vi "HAB Climber.vi"   [LabVIEW 2018]
uses:
  <vilib>/Rock Robotics/SystemInterfaces/DIO/FPGA_DIOChannel.ctl
  <vilib>/Rock Robotics/WPI/ThirdParty/Phoenix-LabVIEW/Motor Controller/Controls/CTRE_Phoenix_MotorControl_ControlMode.ctl
  HAB Climber Global.vi
  <vilib>/Rock Robotics/WPI/Switch/WPI_SwitchOpenLimit.vi
  <vilib>/Rock Robotics/WPI/Counter/WPI_CounterDigitalInputToDigitalSource.vi
  Times/Times Global.vi
  Cargo Intake/Cargo Intake Global.vi
  Controllers/Driver Controller/Driver Controller Global.vi
types:
  T1 = typedef "FPGA_DIOChannel.ctl" = enum8{"DIO 0", "DIO 1", "DIO 2", "DIO 3", "DIO 4", "DIO 5", "DIO 6", "DIO 7", "DIO 8", "DIO 9", "DIO MXP 0", "DIO MXP 1", "DIO MXP 2", "DIO MXP 3", "DIO MXP 4", "DIO MXP 5", "DIO MXP 6", "DIO MXP 7", "DIO MXP 8", "DIO MXP 9", "DIO MXP 10", "DIO MXP 11", "DIO MXP 12", "DIO MXP 13", "DIO MXP 14", "DIO MXP 15", "SPI Port CS1", "SPI Port CS2", "SPI Port CS3", "SPI Port MISO", "SPI Port MOSI", "Invalid"}
  T2 = enum16{"HAB Climber Full Manual Mode", "HAB Climber Manual Mode", "HAB Climber Automated Mode", "HAB Climber Fully Automated Mode"}
  T3 = typedef "WPI_DigitalInputDevRef.ctl" = cluster{"DevStatus":errorcluster, "DIO Channel":T1}
  T4 = typedef "FPGA_CounterEncoderSourceConvertionLVSourceType.ctl" = cluster{"DevStatus":errorcluster, "AnalogTriggerMode?":bool, "DigitalMode":cluster{"DIO Channel":T5}, "AnalogTriggerMode":cluster{"AnalogTriggerIndex":T6, "OutputType":T7}}
  T5 = typedef "FPGA_DIODigitalSourceChannel.ctl" = enum8{"DIO 0", "DIO 1", "DIO 2", "DIO 3", "DIO 4", "DIO 5", "DIO 6", "DIO 7", "DIO 8", "DIO 9", "DIO MXP 0", "DIO MXP 1", "DIO MXP 2", "DIO MXP 3", "DIO MXP 4", "DIO MXP 5", "DIO MXP 6", "DIO MXP 7", "DIO MXP 8", "DIO MXP 9", "DIO MXP 10", "DIO MXP 11", "DIO MXP 12", "DIO MXP 13", "DIO MXP 14", "DIO MXP 15", "SPI Port CS1", "SPI Port CS2", "SPI Port CS3", "SPI Port MISO", "SPI Port MOSI", "Disabled"}
  T6 = typedef "FPGA_AnalogTriggerIndex.ctl" = enum8{"Trig 0", "Trig 1", "Trig 2", "Trig 3", "Trig 4", "Trig 5", "Trig 6", "Trig 7", "Invalid"}
  T7 = typedef "FPGA_AnalogTriggerOutType.ctl" = enum16{"InWindow", "TriggerState", "Rising", "Falling"}
  T8 = typedef "WPI_EncoderDevRef.ctl" = cluster{"DevStatus":errorcluster, "EncoderIndex":T9, "CounterIndex":T10, "DistancePerCount":dbl, "Decoding Type":T11}
  T9 = typedef "FPGA_EncoderIdx.ctl" = enum8{"Enc 0", "Enc 1", "Enc 2", "Enc 3", "Enc 4", "Enc 5", "Enc 6", "Enc 7", "Invalid"}
  T10 = typedef "FPGA_CounterCtrSystemIndex.ctl" = enum8{"Ctr 0", "Ctr 1", "Ctr 2", "Ctr 3", "Ctr 4", "Ctr 5", "Ctr 6", "Ctr 7", "Invalid"}
  T11 = typedef "WPI_EncoderType.ctl" = enum16{"1x", "2x", "4x"}
  T12 = typedef "WPI_SwitchDevRef.ctl" = cluster{"DevStatus":errorcluster, "DIO Channel":T1, "CntIndex":T10, "Normally Closed":bool}
  T13 = typedef "WPI_MotorControlDeviceRef.ctl" = cluster{"DeviceStatus":errorcluster, "Type":T14, "PWM":cluster{"PWM Channel":T15, "DeadBand":T16}, "CAN":cluster{"Device Number":u8, "SetOutput VI Ref":variant, "GetOutput VI Ref":variant, "Enable VI Ref":variant, "Disable VI Ref":variant, "Data":variant}, "Invert":bool, "DIO PWM":cluster{"PWM \"Enable\" Channel":T15, "DIOChannel":T1, "PWM Rate":dbl}}
  T14 = typedef "WPI_MotorControlType.ctl" = enum16{"PWM", "CAN", "DIO PWM"}
  T15 = typedef "FPGA_DIOPWMChannel.ctl" = enum8{"PWM 0", "PWM 1", "PWM 2", "PWM 3", "PWM 4", "PWM 5", "PWM 6", "PWM 7", "PWM 8", "PWM 9", "PWM MXP 0", "PWM MXP 1", "PWM MXP 2", "PWM MXP 3", "PWM MXP 4", "PWM MXP 5", "PWM MXP 6", "PWM MXP 7", "PWM MXP 8", "PWM MXP 9", "Invalid"}
  T16 = typedef "WPI_PWMDeadband.ctl" = cluster{"Name":string, "maxPositivePwm":i32, "minPositivePwm":i32, "centerPwm":i32, "maxNegativePwm":i32, "minNegativePwm":i32, "angularRange":u16}
  T17 = typedef "Control 3.ctl" = dbl
  T18 = typedef "CTRE_Phoenix_MotorControl_ControlMode.ctl" = u16
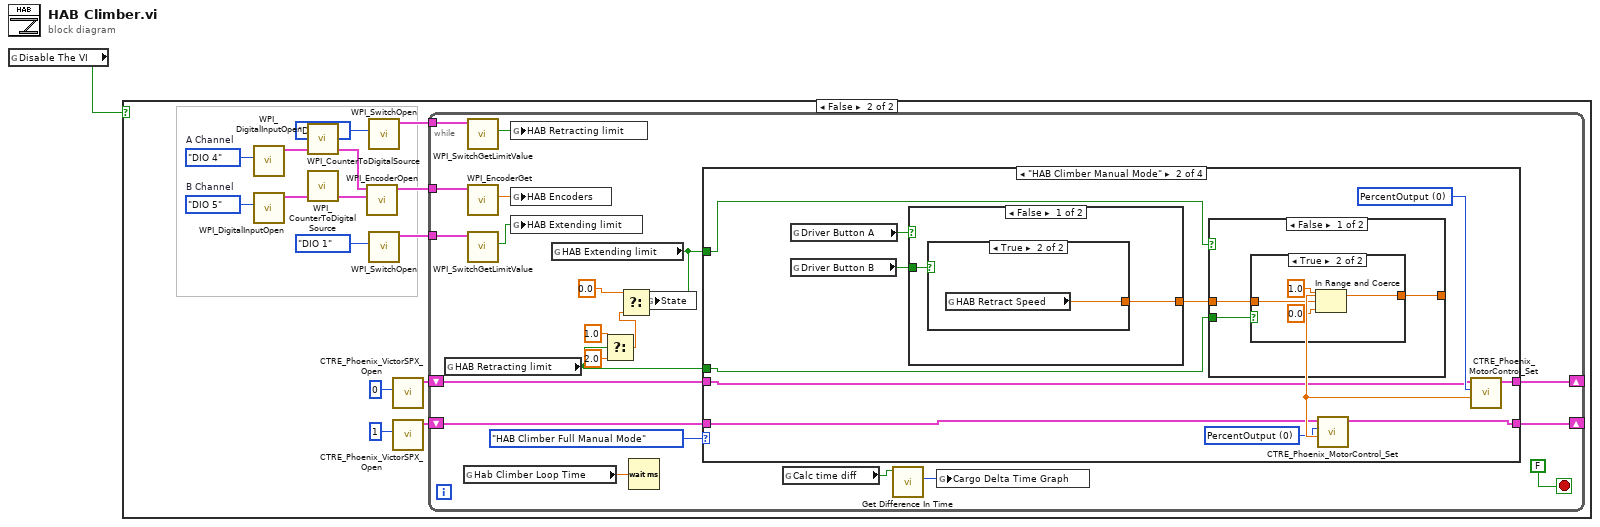
[diagram p0: block diagram]
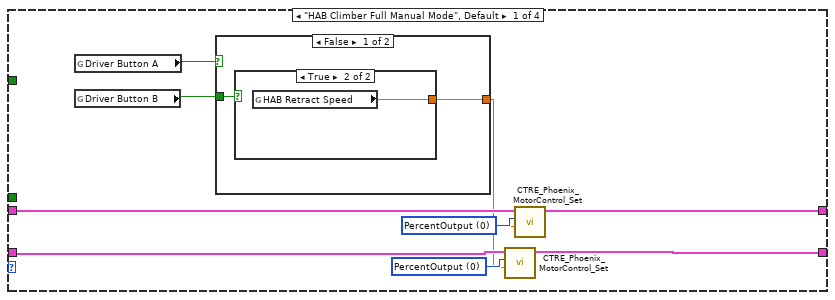
[diagram p3: hidden frame]
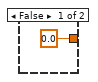
[diagram p4: hidden frame]
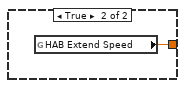
[diagram p5: hidden frame]
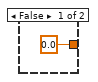
[diagram p6: hidden frame]
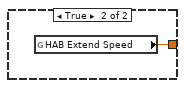
[diagram p7: hidden frame]
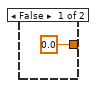
[diagram p8: hidden frame]
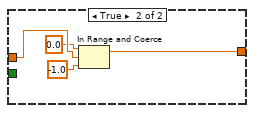
[diagram p9: hidden frame]
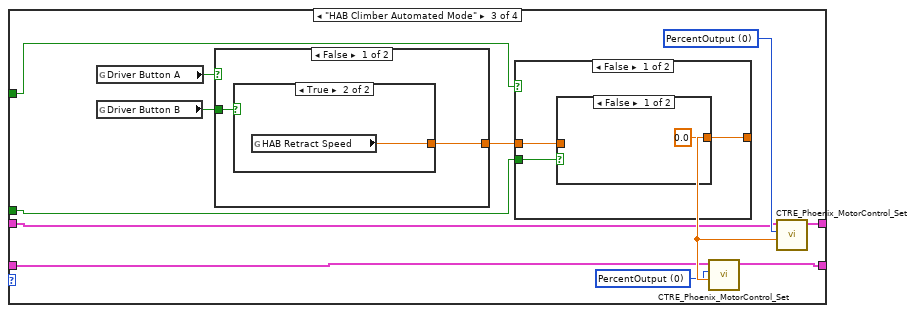
[diagram p10: hidden frame]
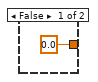
[diagram p11: hidden frame]
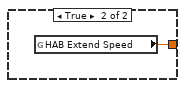
[diagram p12: hidden frame]
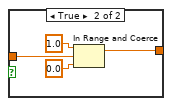
[diagram p13: hidden frame]
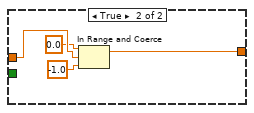
[diagram p14: hidden frame]
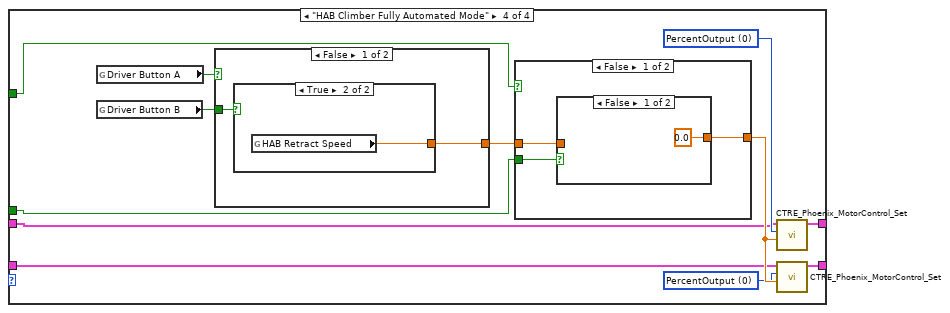
[diagram p15: hidden frame]
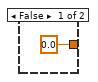
[diagram p16: hidden frame]
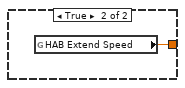
[diagram p17: hidden frame]
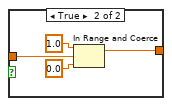
[diagram p18: hidden frame]
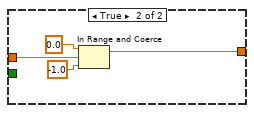
[diagram p19: hidden frame]
diagram:
  n1 = global read "HAB Climber Global.vi" "Disable The VI"() -> (w1:bool)
  n2 = case shown="False" w1 {
    frame True {
    }
    frame False {
      w8 = FPGA_DIOChannel."DIO 5"  # B Channel
      w7 = FPGA_DIOChannel."DIO 4"  # A Channel
      n3 = call <vilib>:"WPI_DigitalInputOpen.vi"("DIO Channel"=w7) -> ("DigitalInputDevRef"=w4:T3)  [unwired: 1 in, 9 out]
      n4 = call <vilib>:"WPI_DigitalInputOpen.vi"("DIO Channel"=w8) -> ("DigitalInputDevRef"=w5:T3)  [unwired: 1 in, 9 out]
      n5 = call-poly <vilib>:"WPI_CounterToDigitalSource.vi"("DigitalInputDevRef"=w4) -> ("Digital Source"=w3:T4)  [unwired: 6 out]
      n6 = call-poly <vilib>:"WPI_CounterToDigitalSource.vi"("DigitalInputDevRef"=w5) -> ("Digital Source"=w6:T4)  [unwired: 6 out]
      n7 = call <vilib>:"WPI_EncoderOpen.vi"("BSource"=w6, "ASource"=w3) -> ("EncoderDevRef"=w2:T8)  [unwired: 6 in, 3 out]
      n8 = call-poly <vilib>:"WPI_SwitchOpen.vi"("DIO Channel"=FPGA_DIOChannel."DIO 2") -> ("SwitchDevRef"=w10:T12)  [unwired: 9 in, 1 out]
      n9 = call-poly <vilib>:"WPI_SwitchOpen.vi"("DIO Channel"=FPGA_DIOChannel."DIO 1") -> ("SwitchDevRef"=w9:T12)  [unwired: 9 in, 1 out]
      n10 = call <vilib>:"CTRE_Phoenix_VictorSPX_Open.vi"("Device Number"=u8 0) -> ("CAN Talon SRX Ref"=w16:T13)  [unwired: 9 in, 1 out]
      n11 = call <vilib>:"CTRE_Phoenix_VictorSPX_Open.vi"("Device Number"=u8 1) -> ("CAN Talon SRX Ref"=w14:T13)  [unwired: 9 in, 1 out]
      n12 = while {
        shift-right: [w33] -> _
        shift-left: w16 -> [w35]
        shift-right: [w32] -> _
        shift-left: w14 -> [w34]
        tunnel: w10 -> [w25]
        tunnel: w9 -> [w24]
        tunnel: w2 -> [w23]
        stop <- FALSE stop-if-true
        n13 = global read "HAB Climber Global.vi" "HAB Retracting limit"() -> (w21:bool)
        n14 = global read "Times Global.vi" "Hab Climber Loop Time"() -> (w38:T17)
        n15 = call <vilib>:"WPI_SwitchGetLimitValue.vi"("SwitchDevRef"=w25) -> ("Switch Pressed"=w19:bool)  [unwired: 8 in, 2 out]
        n16 = call <vilib>:"WPI_EncoderGet.vi"("EncoderDevRef"=w23) -> ("Distance"=w18:dbl)  [unwired: 5 in, 5 out]
        n17 = call <vilib>:"WPI_SwitchGetLimitValue.vi"("SwitchDevRef"=w24) -> ("Switch Pressed"=w20:bool)  [unwired: 8 in, 2 out]
        n18 = global write "HAB Climber Global.vi" "HAB Retracting limit"(w19) -> ()
        n19 = global write "HAB Climber Global.vi" "HAB Encoders"(w18) -> ()
        n20 = global write "HAB Climber Global.vi" "HAB Extending limit"(w20) -> ()
        n21 = global read "HAB Climber Global.vi" "HAB Extending limit"() -> (w22:bool)
        n22 = Select(t=1.0, s=w21, f=2.0 ("t")) -> (s? t:f=w17:dbl)
        n23 = Select(t=0.0, s=w22, f=w17) -> (s? t:f=w29:dbl)
        n24 = Wait (ms)(milliseconds to wait=w38) -> ()  [unwired: 1 out]
        n25 = global write "HAB Climber Global.vi" "State"(w29) -> ()
        n26 = case shown="\"HAB Climber Manual Mode\"" T2."HAB Climber Full Manual Mode" ("Mode") {
          tunnel: w35 -> [w42 w58 w87 w116]
          tunnel: w34 -> [w43 w57 w86 w115]
          tunnel: [w40 w56 w85 w114] -> w33
          tunnel: [w39 w55 w84 w113] -> w32
          tunnel: w22 -> [_ w54 w83 w112]
          tunnel: w21 -> [_ w53 w82 w111]
          frame "HAB Climber Full Manual Mode", Default {
            w44 = T18 0 items=["PercentOutput"=0, "Position"=1, "Velocity"=2, "Current"=3, "Follower"=5, "MotionProfile"=6, "MotionMagic"=7, "MotionProfileArc"=10, "Disabled"=15] ("Control Mode")
            w45 = T18 0 items=["PercentOutput"=0, "Position"=1, "Velocity"=2, "Current"=3, "Follower"=5, "MotionProfile"=6, "MotionMagic"=7, "MotionProfileArc"=10, "Disabled"=15] ("Control Mode")
            n27 = global read "Driver Controller Global.vi" "Driver Button A"() -> (w46:bool)
            n28 = global read "Driver Controller Global.vi" "Driver Button B"() -> (w47:bool)
            n29 = case shown="False" w46 {
              tunnel: w47 -> [w49 _]
              tunnel: [w48 w52] -> w41
              frame False {
                n30 = case shown="True" w49 {
                  tunnel: [0.0 w51] -> w48
                  frame False {
                  }
                  frame True {
                    n31 = global read "HAB Climber Global.vi" "HAB Retract Speed"() -> (w51:dbl)
                  }
                }
              }
              frame True {
                n32 = global read "HAB Climber Global.vi" "HAB Extend Speed"() -> (w52:dbl)
              }
            }
            n33 = call <vilib>:"CTRE_Phoenix_MotorControl_Set.vi"("Output"=w41, "Control Mode"=w44, "PhoenixMotorControlDevRef"=w43) -> ("PhoenixMotorControlDevRef"=w39:T13)  [unwired: 7 in, 1 out]
            n34 = call <vilib>:"CTRE_Phoenix_MotorControl_Set.vi"("Output"=w41, "Control Mode"=w45, "PhoenixMotorControlDevRef"=w42) -> ("PhoenixMotorControlDevRef"=w40:T13)  [unwired: 7 in, 1 out]
          }
          frame "HAB Climber Manual Mode" {
            w59 = T18 0 items=["PercentOutput"=0, "Position"=1, "Velocity"=2, "Current"=3, "Follower"=5, "MotionProfile"=6, "MotionMagic"=7, "MotionProfileArc"=10, "Disabled"=15] ("Control Mode")
            w61 = T18 0 items=["PercentOutput"=0, "Position"=1, "Velocity"=2, "Current"=3, "Follower"=5, "MotionProfile"=6, "MotionMagic"=7, "MotionProfileArc"=10, "Disabled"=15] ("Control Mode")
            n35 = global read "Driver Controller Global.vi" "Driver Button A"() -> (w63:bool)
            n36 = global read "Driver Controller Global.vi" "Driver Button B"() -> (w64:bool)
            n37 = case shown="False" w63 {
              tunnel: w64 -> [w66 _]
              tunnel: [w65 w69] -> w62
              frame False {
                n38 = case shown="True" w66 {
                  tunnel: [0.0 w68] -> w65
                  frame False {
                  }
                  frame True {
                    n39 = global read "HAB Climber Global.vi" "HAB Retract Speed"() -> (w68:dbl)
                  }
                }
              }
              frame True {
                n40 = global read "HAB Climber Global.vi" "HAB Extend Speed"() -> (w69:dbl)
              }
            }
            n41 = case shown="False" w54 {
              tunnel: w62 -> [w71 w81]
              tunnel: [w72 w78] -> w60
              tunnel: w53 -> [w70 _]
              frame False {
                n42 = case shown="True" w70 {
                  tunnel: [0.0 w77] -> w72
                  tunnel: w71 -> [_ w76]
                  frame False {
                  }
                  frame True {
                    n43 = In Range and Coerce(upper limit=1.0, x=w76, lower limit=0.0) -> (coerced(x)=w77:dbl)  [unwired: 1 out]
                  }
                }
              }
              frame True {
                n44 = In Range and Coerce(upper limit=0.0, x=w81, lower limit=-1.0) -> (coerced(x)=w78:dbl)  [unwired: 1 out]
              }
            }
            n45 = call <vilib>:"CTRE_Phoenix_MotorControl_Set.vi"("Output"=w60, "Control Mode"=w59, "PhoenixMotorControlDevRef"=w57) -> ("PhoenixMotorControlDevRef"=w55:T13)  [unwired: 7 in, 1 out]
            n46 = call <vilib>:"CTRE_Phoenix_MotorControl_Set.vi"("Output"=w60, "Control Mode"=w61, "PhoenixMotorControlDevRef"=w58) -> ("PhoenixMotorControlDevRef"=w56:T13)  [unwired: 7 in, 1 out]
          }
          frame "HAB Climber Automated Mode" {
            w88 = T18 0 items=["PercentOutput"=0, "Position"=1, "Velocity"=2, "Current"=3, "Follower"=5, "MotionProfile"=6, "MotionMagic"=7, "MotionProfileArc"=10, "Disabled"=15] ("Control Mode")
            w89 = T18 0 items=["PercentOutput"=0, "Position"=1, "Velocity"=2, "Current"=3, "Follower"=5, "MotionProfile"=6, "MotionMagic"=7, "MotionProfileArc"=10, "Disabled"=15] ("Control Mode")
            n47 = global read "Driver Controller Global.vi" "Driver Button A"() -> (w91:bool)
            n48 = global read "Driver Controller Global.vi" "Driver Button B"() -> (w90:bool)
            n49 = case shown="False" w91 {
              tunnel: w90 -> [w95 _]
              tunnel: [w94 w98] -> w92
              frame False {
                n50 = case shown="True" w95 {
                  tunnel: [0.0 w97] -> w94
                  frame False {
                  }
                  frame True {
                    n51 = global read "HAB Climber Global.vi" "HAB Retract Speed"() -> (w97:dbl)
                  }
                }
              }
              frame True {
                n52 = global read "HAB Climber Global.vi" "HAB Extend Speed"() -> (w98:dbl)
              }
            }
            n53 = case shown="False" w83 {
              tunnel: w92 -> [w100 w110]
              tunnel: [w101 w107] -> w93
              tunnel: w82 -> [w99 _]
              frame False {
                n54 = case shown="False" w99 {
                  tunnel: [0.0 w106] -> w101
                  tunnel: w100 -> [_ w105]
                  frame False {
                  }
                  frame True {
                    n55 = In Range and Coerce(upper limit=1.0, x=w105, lower limit=0.0) -> (coerced(x)=w106:dbl)  [unwired: 1 out]
                  }
                }
              }
              frame True {
                n56 = In Range and Coerce(upper limit=0.0, x=w110, lower limit=-1.0) -> (coerced(x)=w107:dbl)  [unwired: 1 out]
              }
            }
            n57 = call <vilib>:"CTRE_Phoenix_MotorControl_Set.vi"("Output"=w93, "Control Mode"=w88, "PhoenixMotorControlDevRef"=w86) -> ("PhoenixMotorControlDevRef"=w84:T13)  [unwired: 7 in, 1 out]
            n58 = call <vilib>:"CTRE_Phoenix_MotorControl_Set.vi"("Output"=w93, "Control Mode"=w89, "PhoenixMotorControlDevRef"=w87) -> ("PhoenixMotorControlDevRef"=w85:T13)  [unwired: 7 in, 1 out]
          }
          frame "HAB Climber Fully Automated Mode" {
            w117 = T18 0 items=["PercentOutput"=0, "Position"=1, "Velocity"=2, "Current"=3, "Follower"=5, "MotionProfile"=6, "MotionMagic"=7, "MotionProfileArc"=10, "Disabled"=15] ("Control Mode")
            w118 = T18 0 items=["PercentOutput"=0, "Position"=1, "Velocity"=2, "Current"=3, "Follower"=5, "MotionProfile"=6, "MotionMagic"=7, "MotionProfileArc"=10, "Disabled"=15] ("Control Mode")
            n59 = global read "Driver Controller Global.vi" "Driver Button A"() -> (w120:bool)
            n60 = global read "Driver Controller Global.vi" "Driver Button B"() -> (w119:bool)
            n61 = case shown="False" w120 {
              tunnel: w119 -> [w124 _]
              tunnel: [w123 w127] -> w121
              frame False {
                n62 = case shown="True" w124 {
                  tunnel: [0.0 w126] -> w123
                  frame False {
                  }
                  frame True {
                    n63 = global read "HAB Climber Global.vi" "HAB Retract Speed"() -> (w126:dbl)
                  }
                }
              }
              frame True {
                n64 = global read "HAB Climber Global.vi" "HAB Extend Speed"() -> (w127:dbl)
              }
            }
            n65 = case shown="False" w112 {
              tunnel: w121 -> [w129 w139]
              tunnel: [w130 w136] -> w122
              tunnel: w111 -> [w128 _]
              frame False {
                n66 = case shown="False" w128 {
                  tunnel: [0.0 w135] -> w130
                  tunnel: w129 -> [_ w134]
                  frame False {
                  }
                  frame True {
                    n67 = In Range and Coerce(upper limit=1.0, x=w134, lower limit=0.0) -> (coerced(x)=w135:dbl)  [unwired: 1 out]
                  }
                }
              }
              frame True {
                n68 = In Range and Coerce(upper limit=0.0, x=w139, lower limit=-1.0) -> (coerced(x)=w136:dbl)  [unwired: 1 out]
              }
            }
            n69 = call <vilib>:"CTRE_Phoenix_MotorControl_Set.vi"("Output"=w122, "Control Mode"=w118, "PhoenixMotorControlDevRef"=w116) -> ("PhoenixMotorControlDevRef"=w114:T13)  [unwired: 7 in, 1 out]
            n70 = call <vilib>:"CTRE_Phoenix_MotorControl_Set.vi"("Output"=w122, "Control Mode"=w117, "PhoenixMotorControlDevRef"=w115) -> ("PhoenixMotorControlDevRef"=w113:T13)  [unwired: 7 in, 1 out]
          }
        }
        n71 = global read "Cargo Intake Global.vi" "Calc time diff"() -> (w31:bool)
        n72 = call "Get Difference In Time.vi"("Calculate Time Difference"=w31) -> ("Delta Time over Time"=w30:u32)  [unwired: 9 in, 1 out]
        n73 = global write "Times Global.vi" "Cargo Delta Time Graph"(w30) -> ()
      }
    }
  }
